vi "testComMoteurTranslation.vi"() -> ()   [LabVIEW 2023]
uses:
  <vilib>/Instr/_visa.llb/VISA Configure Serial Port (Instr).vi
panel:
  in  "VISA resource name":refnum<visa-resource-name>
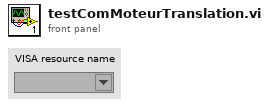
[diagram p1: front panel]
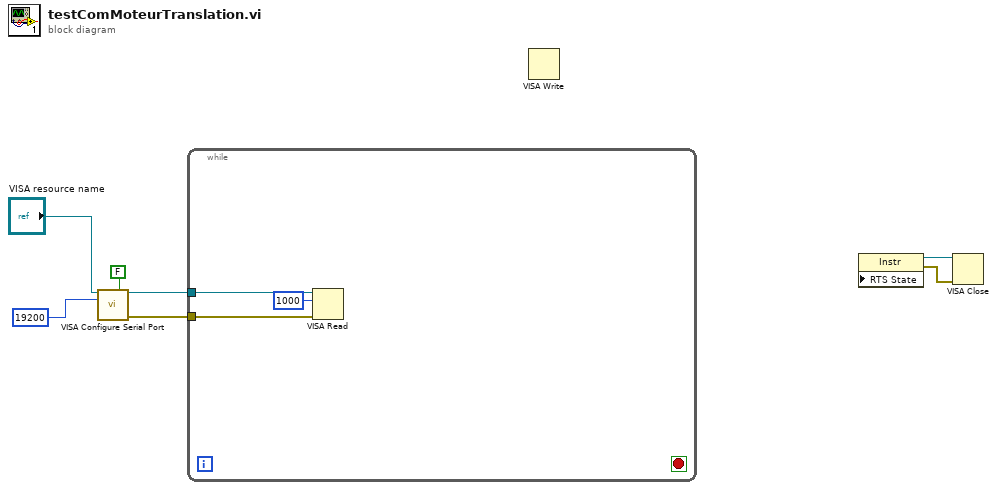
[diagram p0: block diagram]
diagram:
  n1 = call-poly "VISA Configure Serial Port"("VISA resource name"="VISA resource name", "Enable Termination\nChar (T)"=FALSE ("Enable Termination\nChar (T)"), "baud rate (9600)"=u32 19200) -> ("VISA resource name out"=w2:refnum<visa-resource-name>, "error out"=w1:errorcluster)  [unwired: 11 in]
  n2 = while {
    tunnel: w2 -> [w11]
    tunnel: w1 -> [w10]
    stop <- _ stop-if-true
    n3 = VISA Read(VISA resource name=w11, byte count=u32 1000, error in (no error)=w10) -> ()  [unwired: 4 out]
  }
  n4 = VISA Write() -> ()  [unwired: 3 in, 3 out]
  n5 = property class="Instr" props=["RTS State"]() -> (reference=w7:refnum<visa-resource-name>, reference out=w6:refnum<visa-resource-name>, error out=w5:errorcluster)  [unwired: 2 in]
  n6 = VISA Close(VISA resource name=w6, error in (no error)=w5) -> ()  [unwired: 1 out]
